vi "Write hardware.vi"(8 "error in (no error)":errorcluster, 10 "Hardware.lvclass":refnum<class "Target.lvclass">, 11 "Model in":refnum<class "Model.lvclass">) -> (0 "error out":errorcluster, 3 "Model out":refnum<class "Model.lvclass">)   [LabVIEW 2012, in "Model.lvclass"]
uses:
  Model.lvclass
  Target/Target/Target.lvclass
  Model.lvclass/Model.ctl
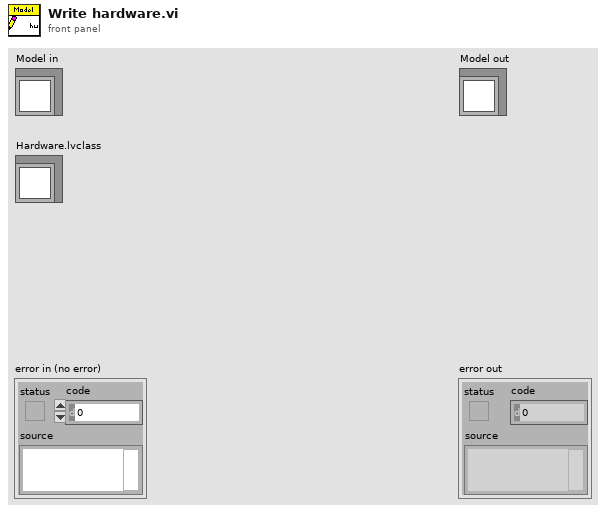
[diagram p1: front panel]
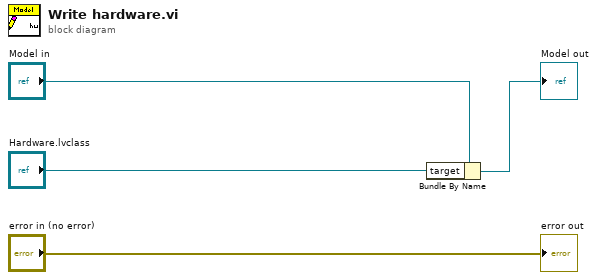
[diagram p0: block diagram]
diagram:
  n1 = Bundle By Name(cluster="Model in", "target"="Hardware.lvclass") -> (→"Model out":refnum<class "Model.lvclass">)
  "error out" <- "error in (no error)"
